vi "play-raster-scan.vi"() -> ()   [LabVIEW 2017]
uses:
  raster-scan-params.ctl
  controls/PI-params.ctl
  controls/boolean_info.ctl
  controls/raster_input_meta_data.ctl
  <vilib>/userdefined/High Color/nirio_resource_hc.ctl
  controls/rasterMetaData.ctl
  <vilib>/Utility/file.llb/Read Delimited Spreadsheet (DBL).vi
  <vilib>/FPGAPlugInAG/cRIO-9082/niLvFpga_Open_cRIO-9082.vi
  <vilib>/rvi/interface/common/dynamic/niFpgaDynamicAddResources.vi
  <vilib>/FPGAPlugInAG/Dynamic/niLvFpga_Reset_Dynamic.vi
  <vilib>/rvi/interface/common/niFpgaWaitOnOcc.vi
  <vilib>/Utility/error.llb/Error Cluster From Error Code.vi
  <vilib>/rvi/errors/niLvFpgaAdjustHostInterfaceError.vi
  <vilib>/FPGAPlugInAG/Dynamic/niLvFpga_Run_Dynamic.vi
  <vilib>/FPGAPlugInAG/Dynamic/niLvFpga_Close_Dynamic.vi
  <userlib>/_matio/level5/Public/Write/Append Data Element.llb/Append Data Element (Anything).vi
  <vilib>/rvi/interface/nirviOpenFPGA/nirviOpenFPGA.xnode
  FPGA Bitfiles/afmimagingcontro_FPGATargetSPARTA_raster-scanning_ejZpyk2O7fU.lvbitx
  <vilib>/rvi/interface/nirviMethod/nirviMethod.xnode
  <vilib>/rvi/interface/nirviReadWriteControl/nirviReadWriteControl.xnode
  <vilib>/rvi/interface/nirviCloseFPGA/nirviCloseFPGA.xnode
  <vilib>/FPGAPlugInAG/Dynamic/niLvFpga_ConfigureFifo_Dynamic.vi
  <vilib>/rvi/errors/niLvFpgaMergeErrorWithErrorCode.vi
  <vilib>/rvi/interface/Simulation/niFpgaSimulationCallBeginRW.vi
  <vilib>/FPGAPlugInAG/Dynamic/niLvFpga_ReadFifo_Dynamic.vi
  NiFpgaLv.dll
  <userlib>/_matio/level5.lvlib
  <vilib>/FPGAPlugInAG/Dynamic/niLvFpga_WriteFifo_Dynamic.vi
  fpga_interface_lib/fpga_interface.lvlib
panel:
  in  "Ring 2":u16(ring) items=["x(k)", "y(k)", "deflection", "u_z"]
  in  "Alert-on-Finish":bool
  in  "do-Dz":bool
  in  "KI_derate":sgl
  in  "ze_sched_thresh":sgl
  out "x":dbl[](graph)
  in  "detrend":bool=TRUE
  out "control":dbl[](graph)
  out "error":dbl[](graph)
  out "InputMetaData":T1
  out "output-meta-data-path":path
  in  "Tab Control":enum32{"Page 1", "Debug"}(tab)
  in  "input-path":path=path "Z:/afm-cs/imaging/raster/5microns/parents/raster_scan_512pix_5mic_01Hz.csv"
  in  "number-of-pixels":i32=512
  out "points_per_line":i32=250000
  out "total_num_points":i32
  in  "raise-constant (init)":sgl
  in  "raise-constant":sgl
  in  "trigger-0":bool
  in  "STOP":bool
  in  "xy-init":fxp<+/-,16,5>[](array[numeric])=[0.0, 0.0]
  in  "Ki-xy":dbl=0.015 format="%#_13g"
  out "ADC-zaxis":sgl
  out "DAC-zaxis":sgl
  in  "xy-bound":sgl=7.0
  out "output-data-path":path
  in  "note-blob":string
  in  "overwrite":bool
  in  "raster-scan-params":T2={"TsTicks"=1600, "Stop"=FALSE, "TOL"=0.3, "ramp-rate"=-0.0002, "z-u-max"=5.0, "PI-params"={"Ki"=0.04, "setpoint"=-0.3}, "Num"=[1.0237086, -2.0434425, 1.0225973, 0.0, 0.0, 0.0, 0.0, 0.0, 0.0], "TF Order"=2, "Den"=[1.0, -1.9961116, 0.998975, 0.0, 0.0, 0.0, 0.0, 0.0, 0.0]} {"ramp-rate" format="%#_5g"; "TOL" format="%#_13g"}
  in  "do_xy_CL":bool=TRUE
  out "boolean errors":T4
  in  "Z-settle-N":i16=10000
  out "Actual Depth":u32
  out "Elements Remaining":u32
  out "size(s)":i32
  out "y iter":i32
  out "nsamps 2":i32
  out "Empty Elements Remaining":u32
  out "(int) y*floor(x/y)":u64
  out "elements left 2":i32=1
  out "x >= y?":bool
  out "writing stopped":bool
  out "size(s) 2":i32
  out "case-selector-feedback":i16
  out "e(0) (threshhold init)":fxp<+/-,16,5>
  out "total-time":dbl
  out "x+1":i32
  out "que timed out?":bool
  out "Error signal (previous line) 2":dbl[](graph)
  out "Waveform Graph":dbl[](graph)
  out "base y_ref (ramp)":dbl[](graph)
  out "base x_ref(triangle wave)":dbl[](graph)
  out "Intensity Graph":dbl[][](graph)
  out "control signal (previous line)":dbl[](graph)
  # "x-axis"
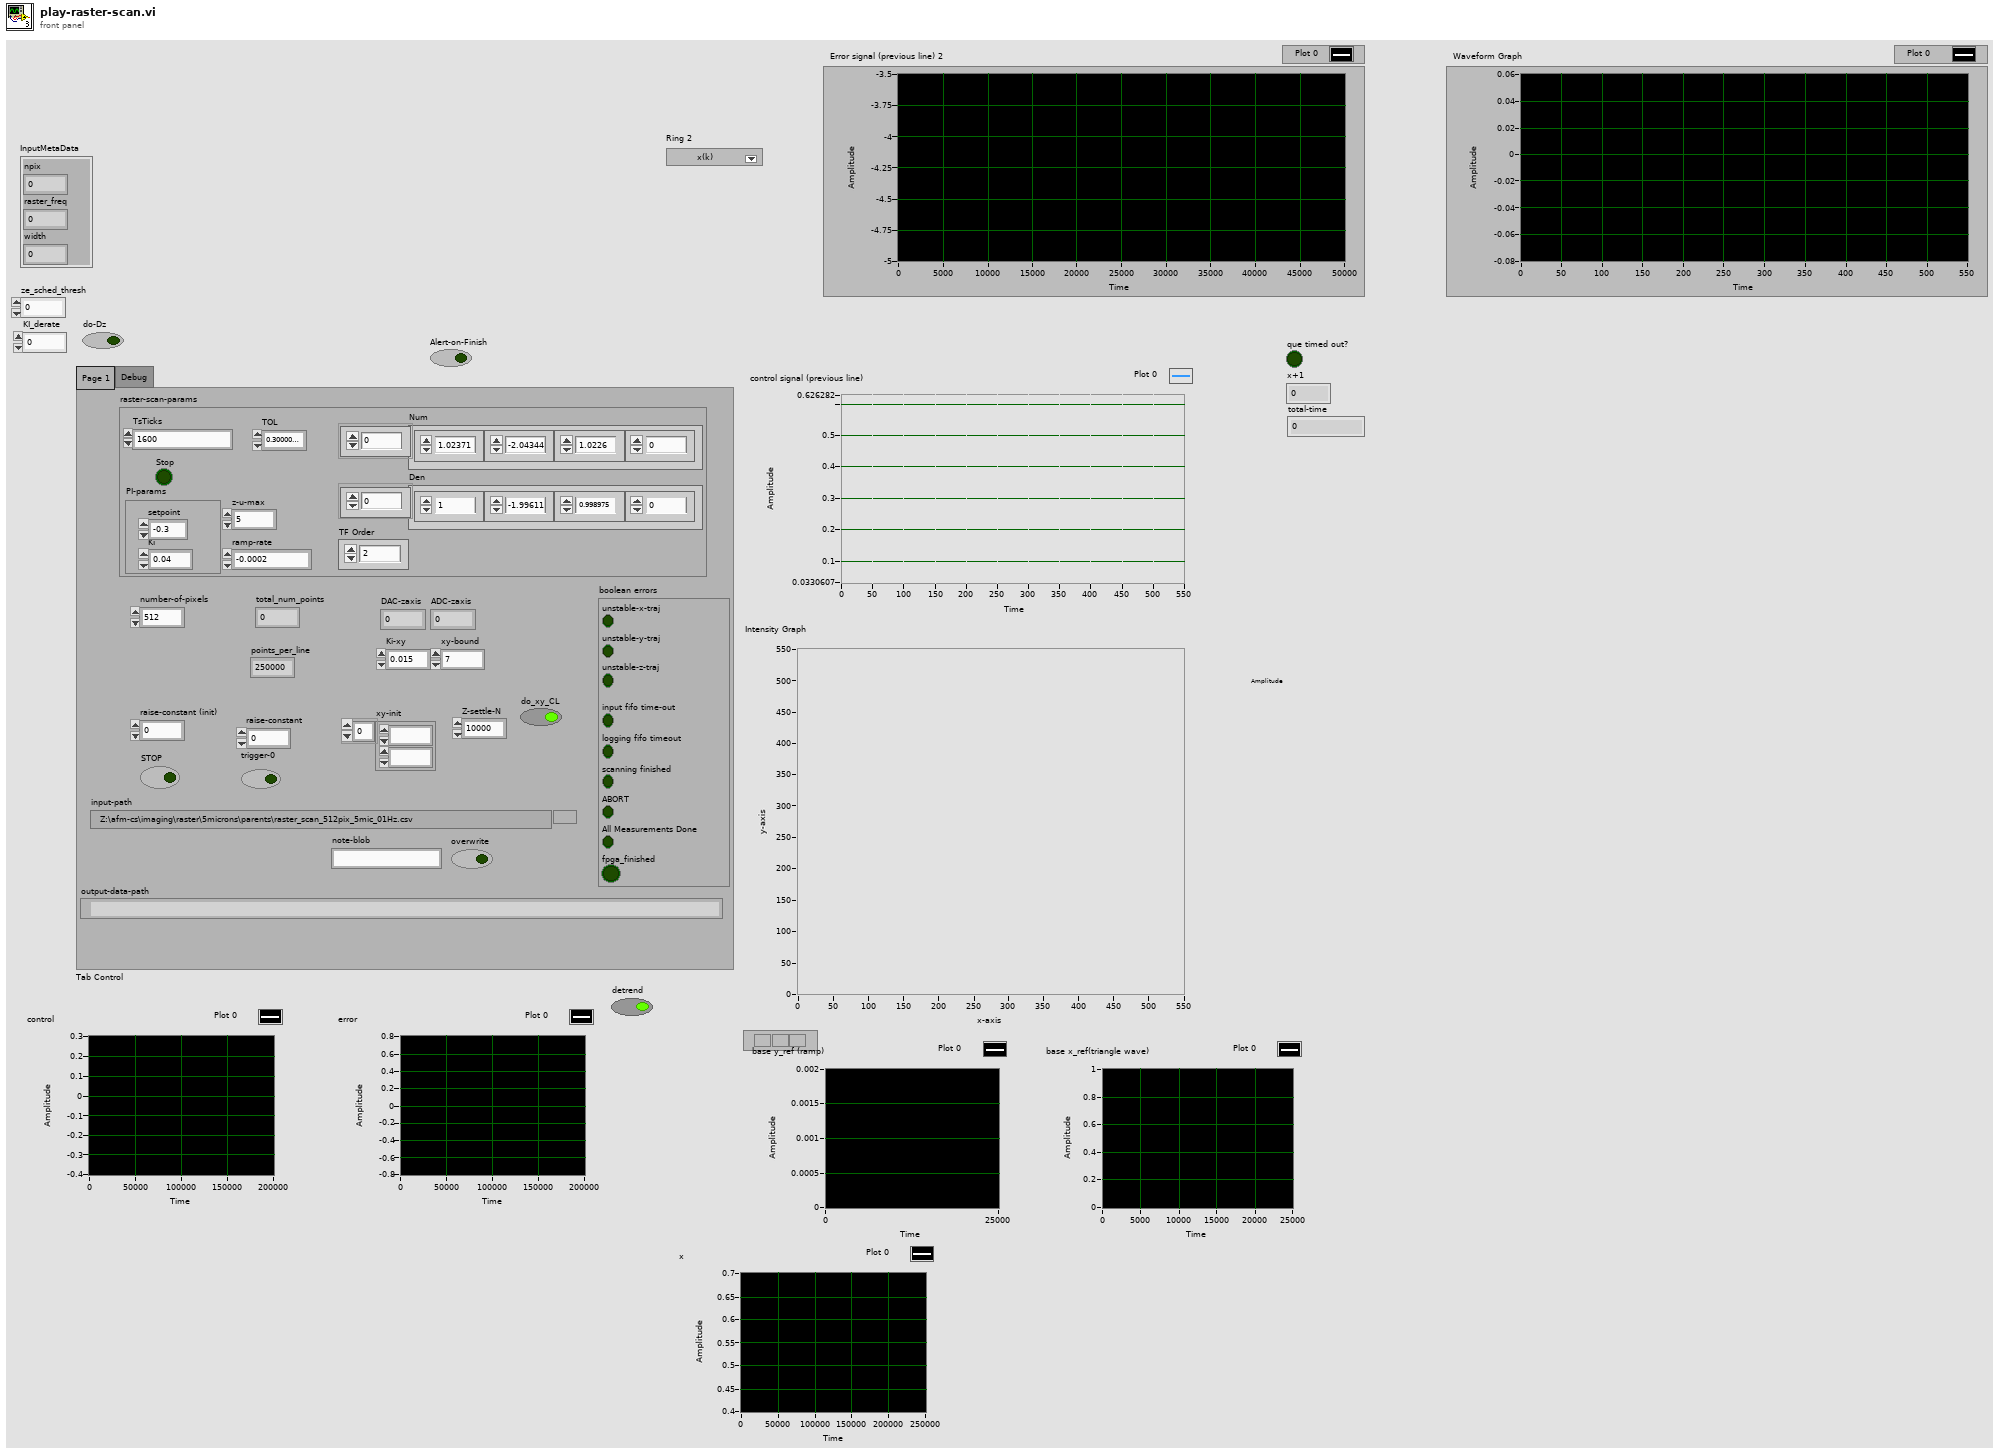
[diagram p1: front panel]
types:
  T1 = typedef "raster_input_meta_data.ctl" = cluster{"npix":dbl, "raster_freq":dbl, "width":dbl}
  T2 = typedef "raster-scan-params.ctl" = cluster{"TsTicks":u32, "Stop":bool, "TOL":sgl, "ramp-rate":sgl, "z-u-max":sgl, "PI-params":T3, "Num":sgl[], "TF Order":i32, "Den":sgl[]}
  T3 = typedef "PI-params.ctl" = cluster{"Ki":sgl, "setpoint":sgl}
  T4 = typedef "boolean_info.ctl" = cluster{"unstable-z-traj":bool, "input fifo time-out":bool, "logging fifo timeout":bool, "scanning finished":bool, "unstable-x-traj":bool, "unstable-y-traj":bool, "ABORT":bool, "All Measurements Done":bool, "fpga_finished":bool}
  T5 = typedef "nirio_resource_hc.ctl" = tag
  T6 = enum16{"open", "replace", "create", "open or create", "replace or create", "replace or create with confirmation"}
  T7 = cluster{"unstable-z-traj":bool, "input fifo time-out":bool, "logging fifo timeout":bool, "scanning finished":bool, "unstable-x-traj":bool, "unstable-y-traj":bool, "ABORT":bool, "All Measurements Done":bool, "fpga_finished":bool}
  T8 = typedef "rasterMetaData.ctl" = cluster{"raster-scan-params":T2, "xy-bound":sgl, "DAC-zaxis":sgl, "ADC-zaxis":sgl, "Ki-xy":dbl, "total_num_points":i32, "points_per_line":i32, "number-of-lines":i32, "number-of-pixels":i32, "raster_meta_in":T1, "Ki-derate":sgl, "ze_sched_thresh":sgl}
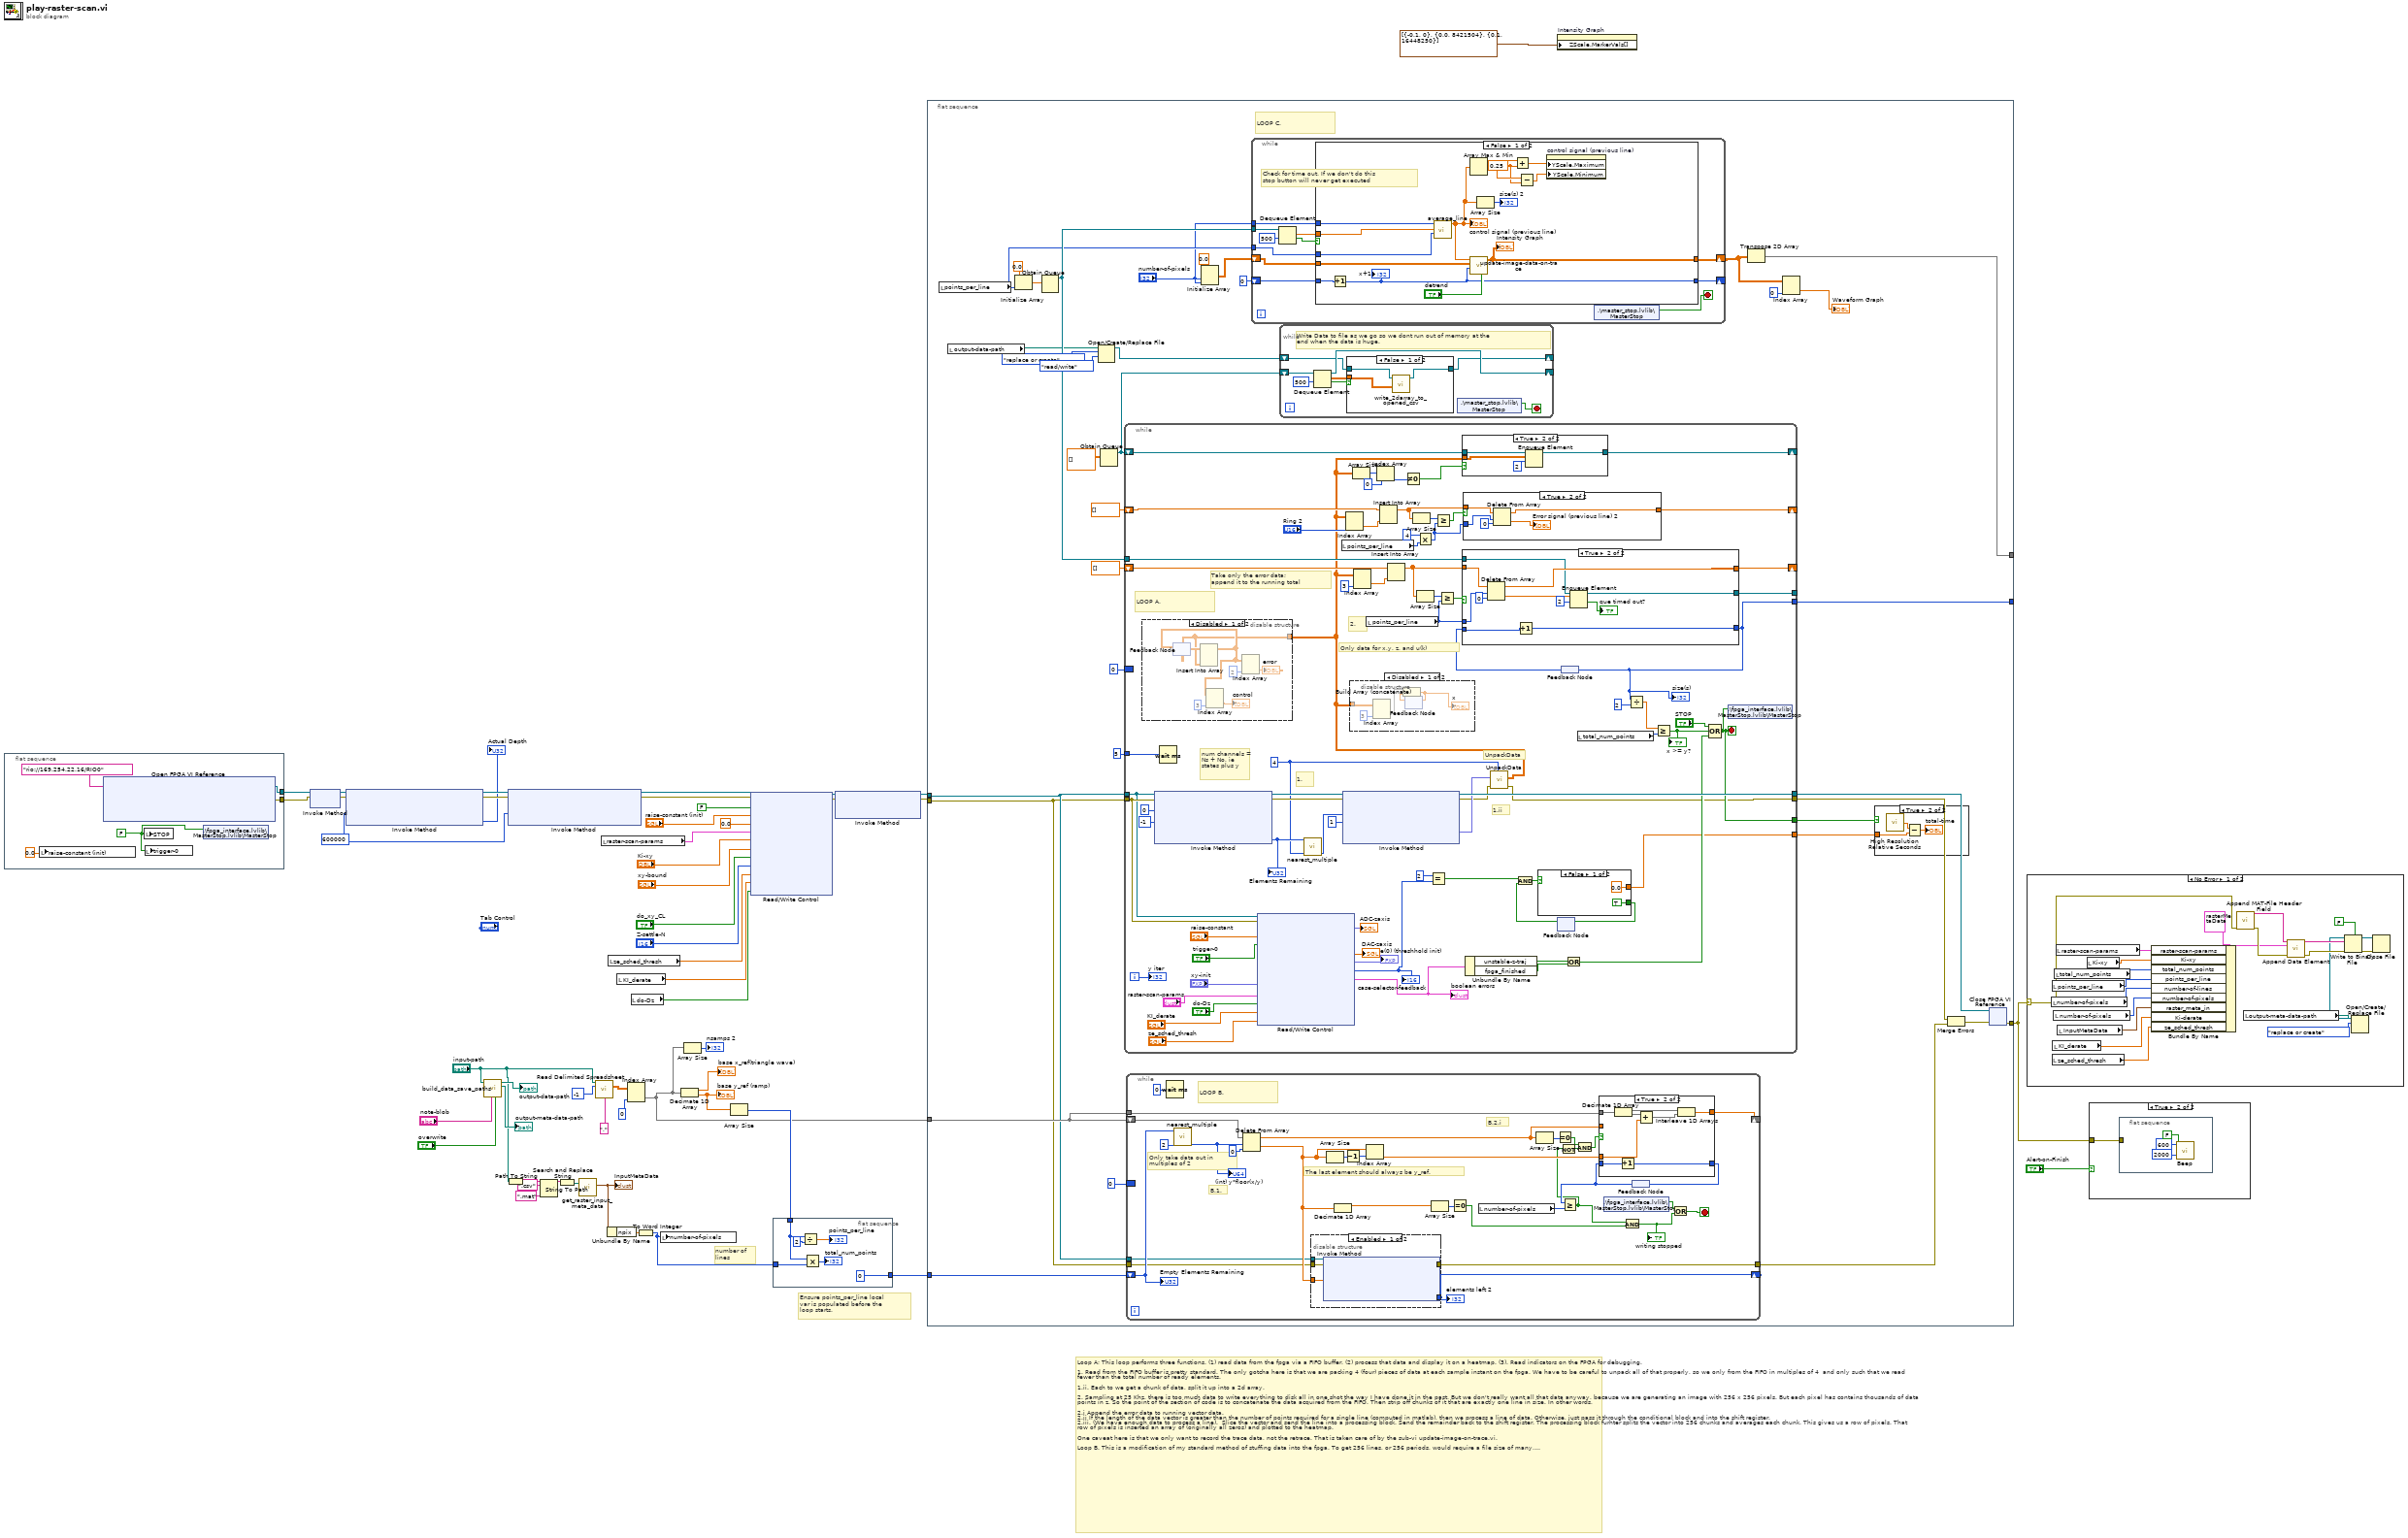
[diagram p0: block diagram]
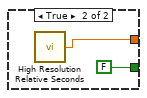
[diagram p11: hidden frame]
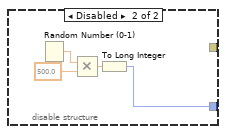
[diagram p14: hidden frame]
diagram:
  w49 = 600000
  # "number of \nlines"
  # "Loop A; This loop performs three functions. (1) read data from the fpga via a FIFO buffer. (2) process that data and display it on a heatmap. (3). Read indicators on the FPGA for debugging.\n\n1. Read from the FIFO buffer is pretty standard. The only gotcha here is that we are packing 4 (four) pieces of data at each sample instant on the fpga. We have to be careful to unpack all of that properly, so we only from the FIFO in multiples of 4  and only such that we read fewer than the total number of ready elements. \n\n1.ii. Each to we get a chunk of data, split it up into a 2d array. \n\n2. Sampling at 25 Khz, there is too much data to write everything to disk all in one shot the way I have done it in the past. But we don't really want all that data anyway, because we are generating an image with 256 x 256 pixels. But each pixel has contains thousands of data points in z. So the point of the section of code is to concatenate the data acquired from the FIFO. Then strip off chunks of it that are exactly one line in size. In other words,\n\n2.i Append the error data to running vector data.\n2.ii If the length of the data vector is greater than the number of points required for a single line (computed in matlab), then we process a line of data. Otherwise, just pass it through the conditional block and into the shift register. \n2.iii. (We have enough data to process a line).  Slice the vector and send the line into a processing block. Send the remainder back to the shift register. The processing block furhter splits the vector into 256 chunks and averages each chunk. This gives us a row of pixels. That row of pixels is inserted an array of (originally all zeros) and plotted to the heatmap.\n\nOne caveat here is that we only want to record the trace data, not the retrace. That is taken care of by the sub-vi update-image-on-trace.vi.\n\nLoop B. This is a modification of my standard method of stuffing data into the fpga. To get 256 lines, or 256 periods, would require a file size of many, many gigibtyes. SO the point here is to only use a single period of the triangle wave and corresponding ramp signal. Everytime we exauhst that data, re-cycle the same data and keep pumping it back in. The one tricky part here is that we have to be careful to shift the original ramp data up by the appropriate amount. We also have to take special care because of how the data is packed from matlab. [x(1), y(1), x(2), y(2)...].\n\nThe first iteration of the loop, we don't push any data in. All we do is get the number of empty elements.\n\nB.1 Each iteration, strip off ' empty elements ' elements from the array and send them to FIFO. \nB.2.i Is the remaining array empty?\nB.2.ii Grab the very last element. We need this"
  # "Ensure points_per_line local\nvar is populated before the\nloop starts."
  n1 = flat-sequence {
    tunnel: [w56] -> w48
    tunnel: [w55] -> w47
    frame #0 {
      w52 = FALSE
      n2 = local write "raise-constant (init)"(0.0) -> ()
      n3 = xnode "Open FPGA VI Reference"("resource name"=T5 "rio://169.254.22.16/RIO0") -> ("FPGA VI Reference Out"=w56:refnum<k20>, "error out"=w55:errorcluster)  [unwired: 1 in]
      n4 = local write "STOP"(w52) -> ()
      n5 = local write "trigger-0"(w52) -> ()
      n6 = shared-variable ".\\fpga_interface.lvlib\\MasterStop.lvlib\\MasterStop"(w52) -> ()  [unwired: 1 in, 1 out]
    }
  }
  n7 = xnode "Invoke Method"("FPGA VI Reference In"=w48, "error in"=w47) -> ("FPGA VI Reference Out"=w44:refnum<k20>, "error out"=w43:errorcluster)
  n8 = xnode "Invoke Method"("FPGA VI Reference In"=w44, "error in"=w43, "Requested Depth"=w49) -> ("FPGA VI Reference Out"=w45:refnum<k20>, "error out"=w46:errorcluster, "Actual Depth"=→"Actual Depth":u32)
  n9 = call "build_data_save_paths.vi"("overwrite"="overwrite", "note-blob"="note-blob", "input-file"="input-path") -> ("output-meta-data-path"=→"output-meta-data-path":path, "output-data-path"=→"output-data-path":path)  [unwired: 5 in, 2 out]
  n10 = Path To String(path="input-path") -> (string=w16:string)
  n11 = xnode "Invoke Method"("FPGA VI Reference In"=w45, "error in"=w46, "Requested Depth"=w49) -> ("FPGA VI Reference Out"=w51:refnum<k20>, "error out"=w50:errorcluster)  [unwired: 1 out]
  n12 = Search and Replace String(input string=w16, search string=".csv", replace string=".mat" ("replace string (\"\")")) -> (result string=w13:string)  [unwired: 5 in, 3 out]
  n13 = String To Path(string=w13) -> (path=w12:path)
  n14 = call "get_raster_input_meta_data.vi"("Path"=w12) -> ("cluster"=w11:T1)  [unwired: 10 in]
  "InputMetaData" <- w11
  n15 = call-poly <vilib>:"Read Delimited Spreadsheet.vi"("file path (dialog if empty)"="input-path", "number of rows (all:-1)"=-1, "delimiter (\\t)"=",") -> ("all rows"=w30:dbl[][])  [unwired: 7 in, 5 out]
  n16 = local read "raster-scan-params"() -> (w8:T2)
  n17 = Unbundle By Name(w11) -> ("npix"=w10:dbl)
  n18 = local read "ze_sched_thresh"() -> (w6:sgl)
  n19 = local read "KI_derate"() -> (w5:sgl)
  n20 = Index Array(array=w30, index (col)=0 ("dimension size")) -> (element=w29:dbl[])  [unwired: 1 in]
  n21 = local read "do-Dz"() -> (w7:bool)
  n22 = To Word Integer(number=w10) -> (16bit integer=w9:i16)
  n23 = local write "number-of-pixels"(w9) -> ()
  n24 = Decimate 1D Array(w29) -> (→"base x_ref(triangle wave)":dbl[], w36:dbl[])
  "base y_ref (ramp)" <- w36
  n25 = Array Size(array=w29) -> (size(s)=→"nsamps 2":i32)
  n26 = Array Size(array=w36) -> (size(s)=w34:i32)
  n27 = xnode "Read/Write Control"("FPGA VI Reference In"=w51, "error in"=w50, "trigger-0"=FALSE ("constant 2 lower"), "raise-constant"="raise-constant (init)", "u(0)"=sgl 0.0, "raster-scan-params"=w8, "Ki-xy"="Ki-xy", "xy-bound"="xy-bound", "do_xy_CL"="do_xy_CL", "Z-settle-N"="Z-settle-N", "ze_sched_thresh"=w6, "KI_derate"=w5, "do-Dz"=w7) -> ("FPGA VI Reference Out"=w26:refnum<k20>, "error out"=w25:errorcluster)
  n28 = flat-sequence {
    tunnel: [0] -> w35
    tunnel: w34 -> [w58]
    tunnel: w9 -> [w61]
    frame #0 {
      n29 = Divide(x=w58, y=2) -> (x/y=→"points_per_line":dbl)
      n30 = Multiply(x=w58, y=w61) -> (x*y=→"total_num_points":i32)
    }
  }
  n31 = xnode "Invoke Method"("FPGA VI Reference In"=w26, "error in"=w25) -> ("FPGA VI Reference Out"=w23:refnum<k20>, "error out"=w24:errorcluster)  [unwired: 1 in]
  n32 = flat-sequence {
    tunnel: [w73] -> _
    tunnel: w23 -> [w82]
    tunnel: w24 -> [w81]
    tunnel: w35 -> [w94]
    tunnel: w29 -> [w83]
    tunnel: [w67] -> _
    tunnel: [w64] -> w2
    frame #0 {
      # "LOOP C."
      n33 = local read "points_per_line"() -> (w79:i32)
      n34 = local read "output-data-path"() -> (w66:path)
      n35 = Initialize Array(0.0 ("element"), w79) -> (w88:dbl[])
      n36 = Obtain Queue(element data type=w88) -> (queue out=w85:refnum<queue>)  [unwired: 4 in, 2 out]
      n37 = Open/Create/Replace File(file path (use dialog)=w66, operation (0:open)=T6."replace or create", access (0:read/write)=enum16{"read/write", "read-only", "write-only"}."read/write") -> (refnum out=w68:refnum<file>)  [unwired: 3 in, 2 out]
      n38 = Obtain Queue(element data type=dbl[][] []) -> (queue out=w71:refnum<queue>)  [unwired: 4 in, 2 out]
      n39 = while {
        tunnel: 5 -> [w212]
        tunnel: w82 -> [w204]
        tunnel: w81 -> [w205]
        tunnel: [w141] -> w76
        tunnel: [w206] -> w77
        shift-right: [w196] -> _
        shift-left: dbl[] [] -> [w194]
        border: 0 ("disabled index (col)") -> [_]
        tunnel: w85 -> [w179]
        tunnel: [w178] -> _
        tunnel: [w146] -> w75
        tunnel: [w170] -> w74
        shift-right: [w164] -> _
        shift-left: w71 -> [w163]
        tunnel: [w162] -> w67
        shift-right: [w149] -> _
        shift-left: dbl[] [] -> [w155]
        i -> [w203]
        stop <- w146 stop-if-true
        w144 = u32 4 ("y")
        # "2."
        # "1.ii"
        # "1."
        # "LOOP A."
        # "Take only the error data;\nappend it to the running total"
        # "num channels = Ns + No, ie states plus y"
        # "Only data for x,y, z, and u(k)"
        # "UnpackData"
        n40 = xnode "Invoke Method"("FPGA VI Reference In"=w204, "error in"=w205, "Number of Elements"=0 ("Timeout (ms)"), "Timeout (ms)"=-1) -> ("FPGA VI Reference Out"=w208:refnum<k20>, "error out"=w209:errorcluster, "Elements Remaining"=w185:u32)  [unwired: 1 out]
        "Elements Remaining" <- w185
        n41 = Wait (ms)(milliseconds to wait=w212) -> ()  [unwired: 1 out]
        n42 = xnode "Read/Write Control"("FPGA VI Reference In"=w204, "error in"=w205, "raise-constant"="raise-constant", "trigger-0"="trigger-0", "xy-init"="xy-init", "raster-scan-params"="raster-scan-params", "do-Dz"="do-Dz", "KI_derate"="KI_derate", "ze_sched_thresh"="ze_sched_thresh") -> ("ADC-zaxis"=→"ADC-zaxis":fxp<+/-,24,5>, "DAC-zaxis"=→"DAC-zaxis":sgl, "e(0) (threshhold init)"=→"e(0) (threshhold init)":fxp<+/-,16,5>, "current-case"=w176:i16, "boolean errors"=w161:T7)  [unwired: 2 out]
        "case-selector-feedback" <- w176
        "boolean errors" <- w161
        n43 = call "nearest_multiple.vi"("numChan"=w144, "N"=w185) -> ("(int) y*floor(x/y)"=w184:u64)  [unwired: 9 in]
        n44 = local read "points_per_line"() -> (w153:i32)
        n45 = xnode "Invoke Method"("FPGA VI Reference In"=w208, "error in"=w209, "Number of Elements"=w184, "Timeout (ms)"=1) -> ("FPGA VI Reference Out"=w206:refnum<k20>, "error out"=w142:errorcluster, "Data"=w143:fxp<+/-,16,5>[])  [unwired: 1 out]
        n46 = local read "points_per_line"() -> (w186:i32)
        n47 = Multiply(x=4, y=w153) -> (x*y=w148:i32)
        n48 = Equal?(x=i16 2, y=w176) -> (x = y?=w174:bool)
        n49 = Unbundle By Name(w161) -> ("unstable-z-traj"=w181:bool, "fpga_finished"=w180:bool)
        n50 = call "UnpackData.vi"("NumChannels"=w144, "error In"=w142, "1D Data In"=w143) -> ("error Out"=w141:errorcluster, "2D Data Out"=w145:dbl[][])  [unwired: 7 in]
        n51 = disable-structure shown="Disabled" {
          disable-tunnel: w145 -> [w224 _]
          frame Disabled {
            n52 = feedback #1(w224) -> (w230:dbl[][])
            n53 = Insert Into Array(array=w230, new element=w224) -> (w225:dbl[][])  [unwired: 2 in]
            n54 = feedback-in #1(w225) -> ()
            n55 = Index Array(array=w225, index (col)=3 ("disabled index (col)")) -> (element=→"control":dbl[])  [unwired: 1 in]
            n56 = Index Array(array=w225, index (col)=2 ("disabled index (col)")) -> (element=→"error":dbl[])  [unwired: 1 in]
          }
          frame Enabled {
          }
        }
        n57 = Index Array(array=w145, index (col)="Ring 2") -> (element=w156:dbl[])  [unwired: 1 in]
        n58 = disable-structure shown="Disabled" {
          disable-tunnel: w145 -> [w222 _]
          frame Disabled {
            n59 = Index Array(array=w222, index (col)=3 ("disabled index (col)")) -> (element=w221:dbl[])  [unwired: 1 in]
            n60 = feedback #2() -> (w220:dbl[])  [unwired: 1 in]
            n61 = Build Array (concatenate)(w221, w220) -> (w219:dbl[])
            "x" <- w219
            n62 = feedback-in #2(w219) -> ()
          }
          frame Enabled {
          }
        }
        n63 = Array Size(array=w145) -> (size(s)=w168:i32[])
        n64 = Index Array(array=w145, index (col)=3 ("disabled index (col)")) -> (element=w193:dbl[])  [unwired: 1 in]
        n65 = Index Array(array=w168, index=0) -> (element=w166:i32)
        n66 = Insert Into Array(array=w155, new element=w156) -> (w150:dbl[])  [unwired: 1 in]
        n67 = Insert Into Array(array=w194, new element=w193) -> (w169:dbl[])  [unwired: 1 in]
        n68 = Not Equal To 0?(x=w166) -> (x != 0?=w165:bool)
        n69 = Array Size(array=w150) -> (size(s)=w154:i32)
        n70 = Array Size(array=w169) -> (size(s)=w195:i32)
        n71 = Greater Or Equal?(x=w154, y=w148) -> (x >= y?=w151:bool)
        n72 = Greater Or Equal?(x=w195, y=w186) -> (x >= y?=w192:bool)
        n73 = case shown="True" w165 {
          tunnel: w163 -> [w231 w235]
          tunnel: w145 -> [_ w233]
          tunnel: [w231 w232] -> w164
          frame False {
          }
          frame True {
            n74 = Enqueue Element(queue=w235, element=w233, timeout in ms (-1)=2) -> (queue out=w232:refnum<queue>)  [unwired: 1 in, 2 out]
          }
        }
        n75 = case shown="True" w151 {
          tunnel: w150 -> [w213 w218]
          tunnel: [w213 w215] -> w149
          tunnel: w148 -> [_ w216]
          frame False {
          }
          frame True {
            n76 = Delete From Array(array=w218, length=w216, index=0) -> (deleted portion=→"Error signal (previous line) 2":dbl[], array with subset deleted=w215:dbl[])
          }
        }
        n77 = feedback #3() -> (w172:bool)  [unwired: 1 in]
        n78 = And(x=w174, y=w172) -> (x .and. y?=w175:bool)
        n79 = case shown="False" w175 {
          tunnel: [TRUE FALSE] -> w173
          tunnel: [0.0 ("relative seconds") w238] -> w170
          frame False {
          }
          frame True {
            n80 = call <vilib>:"High Resolution Relative Seconds.vi"() -> ("relative seconds"=w238:dbl)
          }
        }
        n81 = feedback-in #3(w173) -> ()
        n82 = feedback #4() -> (w191:i32)
        n83 = case shown="True" w192 {
          tunnel: [w242 w251] -> w196
          tunnel: w169 -> [w242 w253]
          tunnel: w191 -> [w241 w250]
          tunnel: [w241 w249] -> w162
          tunnel: w186 -> [_ w248]
          tunnel: w179 -> [w240 w246]
          tunnel: [w240 w245] -> w178
          frame False {
          }
          frame True {
            n84 = Delete From Array(array=w253, length=w248, index=0) -> (deleted portion=w247:dbl[], array with subset deleted=w251:dbl[])
            n85 = Increment(x=w250) -> (x+1=w249:i32)
            n86 = Enqueue Element(queue=w246, element=w247, timeout in ms (-1)=2) -> (queue out=w245:refnum<queue>, timed out?=→"que timed out?":bool)  [unwired: 1 in, 1 out]
          }
        }
        "size(s)" <- w162
        n87 = feedback-in #4(w162) -> ()
        n88 = Or(x=w181, y=w180) -> (x .or. y?=w187:bool)
        n89 = local read "total_num_points"() -> (w190:i32)
        n90 = Divide(x=w162, y=2) -> (x/y=w183:dbl)
        n91 = Greater Or Equal?(x=w183, y=w190) -> (x >= y?=w188:bool)
        "x >= y?" <- w188
        n92 = Compound Arithmetic op=OR("STOP", w188, w187) -> (w146:bool)
        n93 = shared-variable ".\\fpga_interface.lvlib\\MasterStop.lvlib\\MasterStop"(w146) -> ()  [unwired: 1 in, 1 out]
        "y iter" <- w203
      }
      n94 = while {
        shift-right: [w283] -> _
        shift-left: w94 -> [w279]
        shift-right: [w272] -> _
        shift-left: w83 -> [w284]
        tunnel: w83 -> [w270]
        tunnel: [w276] -> w95
        tunnel: w82 -> [w268]
        tunnel: w81 -> [w267]
        border: 0 ("Timeout (ms)") -> [_]
        stop <- w280 stop-if-true
        # "B.2.i"
        # "B.1."
        # "LOOP B."
        # "Only take data out in \nmultiples of 2"
        # "The last element should always be y_ref."
        n95 = Wait (ms)(milliseconds to wait=0) -> ()  [unwired: 1 out]
        n96 = call "nearest_multiple.vi"("numChan"=u32 2 ("Empty Elements Remaining"), "N"=w279) -> ("(int) y*floor(x/y)"=w278:u64)  [unwired: 9 in]
        "(int) y*floor(x/y)" <- w278
        n97 = Delete From Array(array=w284, length=w278, index=0) -> (deleted portion=w273:dbl[], array with subset deleted=w271:dbl[])
        n98 = disable-structure shown="Enabled" {
          disable-tunnel: [w299 w300] -> w283
          disable-tunnel: w273 -> [w298 _]
          disable-tunnel: [w297 _] -> w276
          disable-tunnel: w268 -> [w296 _]
          disable-tunnel: w267 -> [w295 _]
          frame Enabled {
            n99 = xnode "Invoke Method"("FPGA VI Reference In"=w296, "error in"=w295, "Data"=w298) -> ("error out"=w297:errorcluster, "Empty Elements Remaining"=w299:u32)  [unwired: 1 in, 1 out]
          }
          frame Disabled {
            n100 = Random Number (0-1)() -> (number: 0 to 1=w303:dbl)
            n101 = Multiply(x=w303, y=500.0) -> (x*y=w301:dbl)
            n102 = To Long Integer(number=w301) -> (32bit integer=w300:i32)
          }
        }
        "elements left 2" <- w283
        n103 = Array Size(array=w273) -> (size(s)=w274:i32)
        n104 = Decimate 1D Array(w273) -> (w259:dbl[])  [unwired: 1 out]
        n105 = Decrement(x=w274) -> (x-1=w275:i32)
        n106 = Index Array(array=w273, index=w275) -> (element=w269:dbl)
        n107 = Array Size(array=w259) -> (size(s)=w261:i32)
        n108 = Equal To 0?(x=w261) -> (x = 0?=w260:bool)
        n109 = local read "number-of-pixels"() -> (w265:i32)
        n110 = Array Size(array=w271) -> (size(s)=w281:i32)
        n111 = Equal To 0?(x=w281) -> (x = 0?=w258:bool)
        n112 = shared-variable ".\\fpga_interface.lvlib\\MasterStop.lvlib\\MasterStop"() -> (w254:bool)  [unwired: 1 in, 1 out]
        n113 = feedback #5() -> (w263:i32)
        n114 = Greater Or Equal?(x=w263, y=w265) -> (x >= y?=w256:bool)
        n115 = Not(x=w256) -> (.not. x?=w257:bool)
        n116 = And(x=w258, y=w257) -> (x .and. y?=w255:bool)
        n117 = case shown="True" w255 {
          tunnel: [w286 w289] -> w272
          tunnel: w271 -> [w286 _]
          tunnel: w270 -> [_ w294]
          tunnel: w269 -> [_ w292]
          tunnel: [w285 w288] -> w264
          tunnel: w263 -> [w285 w287]
          frame False {
          }
          frame True {
            n118 = Decimate 1D Array(w294) -> (w291:dbl[], w293:dbl[])
            n119 = Increment(x=w287) -> (x+1=w288:i32)
            n120 = Add(x=w293, y=w292) -> (x+y=w290:dbl[])
            n121 = Interleave 1D Arrays(w291, w290) -> (w289:dbl[])
          }
        }
        n122 = And(x=w256, y=w260) -> (x .and. y?=w262:bool)
        "writing stopped" <- w262
        n123 = feedback-in #5(w264) -> ()
        n124 = Or(x=w254, y=w262) -> (x .or. y?=w280:bool)
        "Empty Elements Remaining" <- w279
      }
      n125 = Initialize Array(0.0 ("element"), "number-of-pixels", "number-of-pixels") -> (w87:dbl[][])
      n126 = while {
        shift-right: [w123] -> w84
        shift-left: w87 -> [w122]
        shift-right: [w120] -> _
        shift-left: 0 ("disabled index (col)") -> [w121]
        tunnel: w79 -> [w119]
        tunnel: w85 -> [w118]
        tunnel: "number-of-pixels" -> [w114]
        stop <- w113 stop-if-true
        # "Check for time out. If we don't do this\nstop button will never get executed"
        n127 = Dequeue Element(queue=w118, timeout in ms (-1)=500) -> (element=w117:dbl[], timed out?=w115:bool)  [unwired: 1 in, 2 out]
        n128 = case shown="False" w115 {
          tunnel: [w138 w139] -> w123
          tunnel: w122 -> [w137 w139]
          tunnel: w121 -> [w136 w140]
          tunnel: [w125 w140] -> w120
          tunnel: w119 -> [w135 _]
          tunnel: w117 -> [w134 _]
          tunnel: w114 -> [w132 _]
          frame False {
            w126 = 0.25
            n129 = Increment(x=w136) -> (x+1=w125:i32)
            "x+1" <- w125
            n130 = call "average_line.vi"("data-pts-per-line"=w135, "raw-data-row"=w134, "number-of-pixels"=w132) -> ("avg-data-row"=w124:dbl[])  [unwired: 8 in]
            "control signal (previous line)" <- w124
            n131 = Array Max & Min(array=w124) -> (max value=w130:dbl, min value=w127:dbl)  [unwired: 2 out]
            n132 = call "update-image-data-on-trace.vi"("detrend"="detrend", "iterator"=w125, "master-image-data-n"=w137, "avg-data-row"=w124) -> ("master-image-data-out"=w138:dbl[][])  [unwired: 7 in]
            "Intensity Graph" <- w138
            n133 = Array Size(array=w124) -> (size(s)=→"size(s) 2":i32)
            n134 = Add(x=w130, y=w126) -> (x+y=w129:dbl)
            n135 = Subtract(x=w127, y=w126) -> (x-y=w128:dbl)
            n136 = property on="control signal (previous line)" class="WFGraph (strict)"("YScale.Maximum"=w129, "YScale.Minimum"=w128) -> ()  [unwired: 2 in, 2 out]
          }
          frame True {
          }
        }
        n137 = shared-variable ".\\master_stop.lvlib\\MasterStop"() -> (w113:bool)  [unwired: 1 in, 1 out]
      }
      n138 = while {
        shift-right: [w101] -> _
        shift-left: w71 -> [w102]
        shift-right: [w99] -> _
        shift-left: w68 -> [w100]
        stop <- w98 stop-if-true
        # "Write Data to file as we go so we dont run out of memory at the \nend when the data is huge."
        n139 = Dequeue Element(queue=w102, timeout in ms (-1)=500) -> (queue out=w101:refnum<queue>, element=w103:dbl[][], timed out?=w104:bool)  [unwired: 1 in, 1 out]
        n140 = case shown="False" w104 {
          tunnel: w103 -> [w106 _]
          tunnel: w100 -> [w108 w109]
          tunnel: [w107 w109] -> w99
          frame False {
            n141 = call "write_2darray_to_opened_csv.vi"("Data_in"=w106, "file_ref_in"=w108) -> ("file_ref_out"=w107:refnum<file>)  [unwired: 9 in]
          }
          frame True {
          }
        }
        n142 = shared-variable ".\\master_stop.lvlib\\MasterStop"() -> (w98:bool)  [unwired: 1 in, 1 out]
      }
      n143 = Transpose 2D Array(2D array=w84) -> (transposed array=w73:dbl[][])
      n144 = Index Array(array=w84, index (col)=0 ("disabled index (col)")) -> (element=→"Waveform Graph":dbl[])  [unwired: 1 in]
      n145 = case shown="True" w75 {
        tunnel: w74 -> [_ w112]
        frame False {
        }
        frame True {
          n146 = call <vilib>:"High Resolution Relative Seconds.vi"() -> ("relative seconds"=w111:dbl)
          n147 = Subtract(x=w111, y=w112) -> (x-y=→"total-time":dbl)
        }
      }
      n148 = Merge Errors(w76, w95) -> (w65:errorcluster)
      n149 = xnode "Close FPGA VI Reference"("FPGA VI Reference In"=w77, "error in"=w65) -> ("error out"=w64:errorcluster)
    }
  }
  n150 = property on="Intensity Graph" class="IntGraph (strict)"("ZScale.MarkerVals[]"=cluster{dbl, u32}[] [{-0.1, 0}, {0.0, 8421504}, {0.1, 16448250}] ("Z Scale.Marker Values[]")) -> ()  [unwired: 2 in, 2 out]
  n151 = case shown="No Error" w2 {
    selector: w2 -> [w314 _]
    frame No Error {
      n152 = local read "number-of-pixels"() -> (w308:i32)
      n153 = local read "points_per_line"() -> (w309:i32)
      n154 = local read "ze_sched_thresh"() -> (w304:sgl)
      n155 = local read "KI_derate"() -> (w305:sgl)
      n156 = local read "number-of-pixels"() -> (w307:i32)
      n157 = local read "total_num_points"() -> (w310:i32)
      n158 = local read "raster-scan-params"() -> (w312:T2)
      n159 = local read "InputMetaData"() -> (w306:T1)
      n160 = local read "Ki-xy"() -> (w311:dbl)
      n161 = Bundle By Name(cluster=T8 {"raster-scan-params"={"TsTicks"=1600, "Stop"=TRUE, "TOL"=0.3, "ramp-rate"=-5e-05, "z-u-max"=5.0, "PI-params"={"Ki"=0.01, "setpoint"=0.0}, "Num"=[1.0, 0.0, 0.0, 0.0, 0.0, 0.0, 0.0, 0.0, 0.0], "TF Order"=3, "Den"=[1.0, 0.0, 0.0, 0.0, 0.0, 0.0, 0.0, 0.0, 0.0]}, "xy-bound"=7.0, "DAC-zaxis"=0.0, "ADC-zaxis"=0.0, "Ki-xy"=0.01, "total_num_points"=0, "points_per_line"=250000, "number-of-lines"=256, "number-of-pixels"=256, "raster_meta_in"={"npix"=0.0, "raster_freq"=0.0, "width"=0.0}, "Ki-derate"=0.01, "ze_sched_thresh"=0.0} ("Cluster"), "raster-scan-params"=w312, "Ki-xy"=w311, "total_num_points"=w310, "points_per_line"=w309, "number-of-lines"=w308, "number-of-pixels"=w307, "raster_meta_in"=w306, "Ki-derate"=w305, "ze_sched_thresh"=w304) -> (w313:T8)
      n162 = call <userlib>:"Append MAT-File Header Field.vi"("error"=w314) -> ("result string"=w325:string, "error out"=w319:errorcluster)  [unwired: 13 in]
      n163 = local read "output-meta-data-path"() -> (w316:path)
      n164 = call-poly <userlib>:"Append Data Element.vi"("initial string"=w325, "data"=w313, "error in (no error)"=w319) -> ("result string"=w323:string, "error out"=w324:errorcluster)  [unwired: 11 in]
      n165 = Open/Create/Replace File(file path (use dialog)=w316, operation (0:open)=T6."replace or create") -> (refnum out=w318:refnum<file>)  [unwired: 4 in, 2 out]
      n166 = Write to Binary File(file (use dialog)=w318, data=w323, error in=w324, 5:FALSE ("prepend array or string size? (T)")) -> (refnum out=w320:refnum<file>, error out=w321:errorcluster)  [unwired: 2 in, 1 out]
      n167 = Close File(refnum=w320, error in=w321) -> ()  [unwired: 2 out]
    }
    frame Error {
    }
  }
  n168 = case shown="True" "Alert-on-Finish" {
    tunnel: w2 -> [_ w326]
    frame False {
    }
    frame True {
      n169 = flat-sequence {
        tunnel: w326 -> [_]
        frame #0 {
          n170 = call <vilib>:"Beep.vi"("use system alert? (T)"=FALSE, "duration (msec)"=u32 2000, "frequency (Hz)"=u32 600) -> ()  [unwired: 9 in]
        }
      }
    }
  }
